vi "MCLB_FocusNameArray_Tests.vi"(11 "error in":errorcluster) -> (15 "error out":errorcluster)   [LabVIEW 2016, in "DronaTest.lvlib"]
uses:
  DronaTest.lvlib
  APIs/Stimulus/ControlValue/typedef/Name&Occurrence.ctl
  APIs/Stimulus/ControlValue/SetValueAuto.vi
  APIs/Stimulus/ControlValue/Controls/MC Listbox/SetValueByArrayName.vi
  APIs/Assert/AssertControlValue/Controls/MC Listbox/AssertValueByArrayName.vi
  <vilib>/addons/_JKI Toolkits/Caraya/classes/Assert/Assert Error.vi
  <vilib>/addons/_JKI Toolkits/Caraya/classes/Assert/Assert Equal Value_Variant.vi
  <vilib>/addons/_JKI Toolkits/Caraya/classes/Test/Test.lvclass
  Drona.lvlib
  <vilib>/SLL Toolkit/SLL Debug/SLL Debug.lvlib
  APIs/Stimulus/ControlValue/ControlValue.lvlib
  <vilib>/addons/_JKI Toolkits/Caraya/classes/Assert/Assert.lvclass
  APIs/Stimulus/ControlValue/Controls/MC Listbox/StimulusMCListbox.lvlib
  APIs/Assert/AssertControlValue/Controls/MC Listbox/AssertMCListbox.lvlib
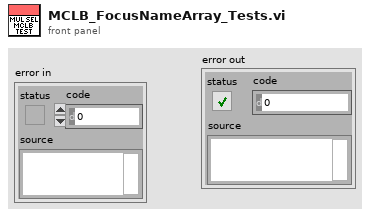
[diagram p1: front panel]
types:
  T1 = typedef "Drona.lvlib/ControlValue.lvlib/Name&Occurrence.ctl" = cluster{"ItemName":string, "Occurrence":i32}
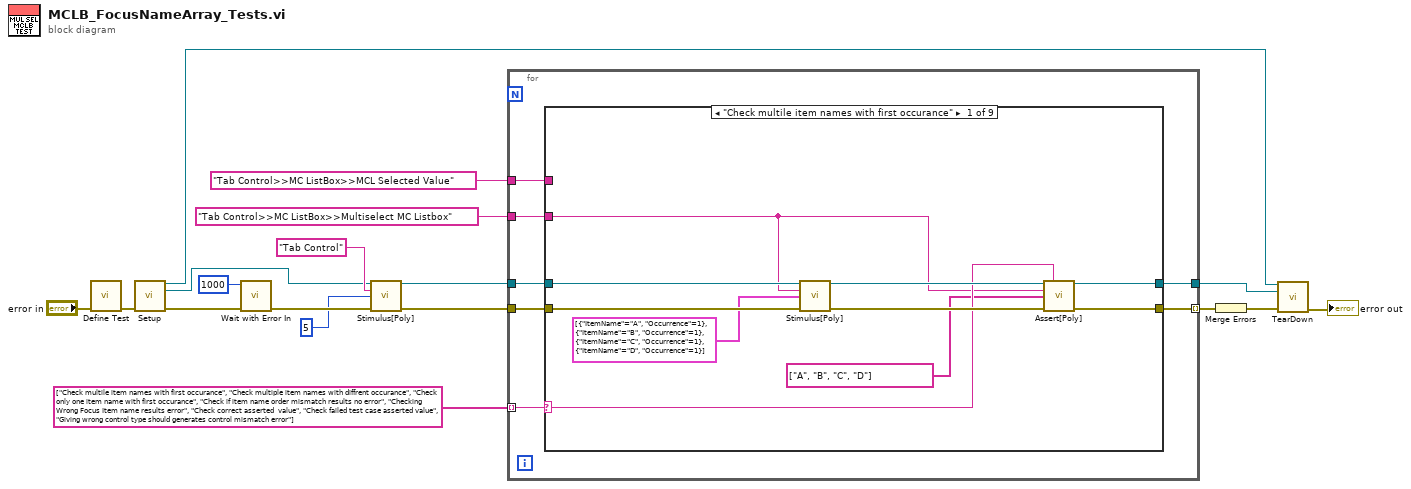
[diagram p0: block diagram]
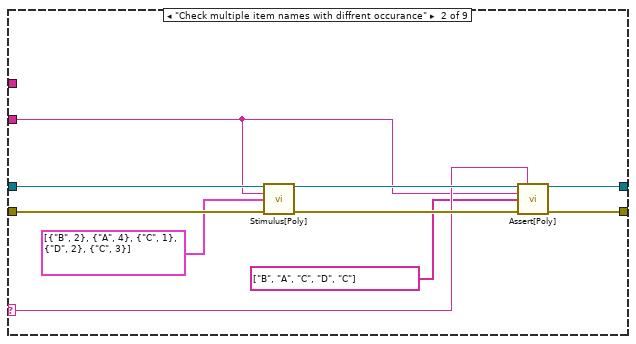
[diagram p2: hidden frame]
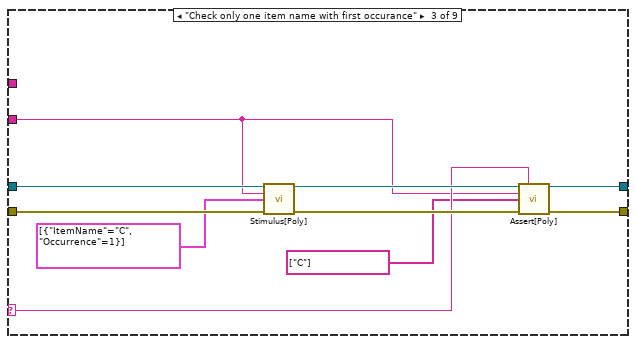
[diagram p3: hidden frame]
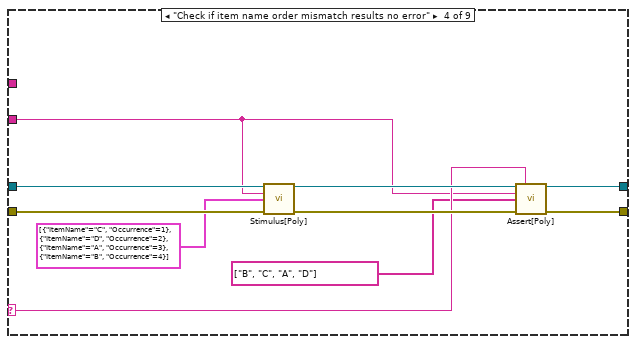
[diagram p4: hidden frame]
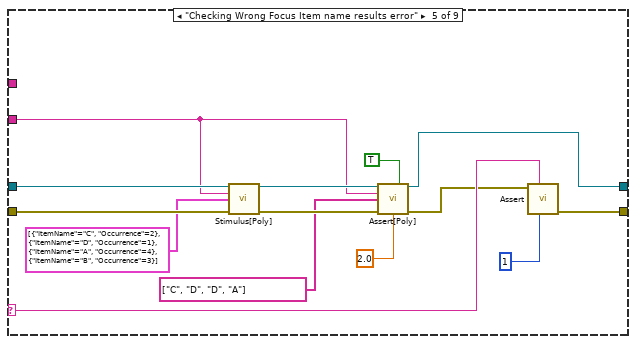
[diagram p5: hidden frame]
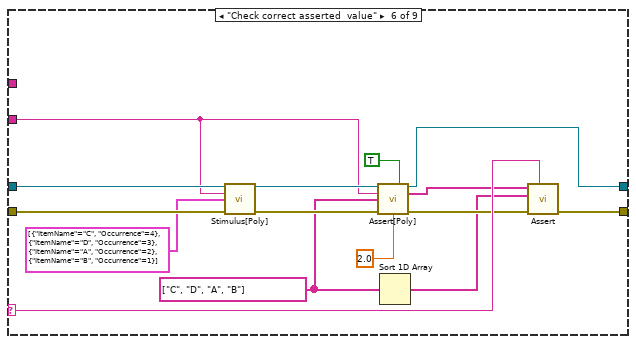
[diagram p6: hidden frame]
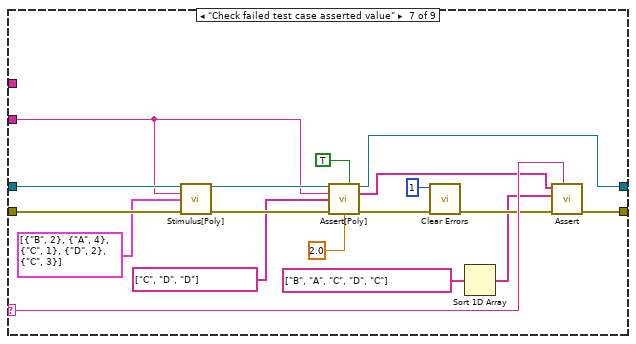
[diagram p7: hidden frame]
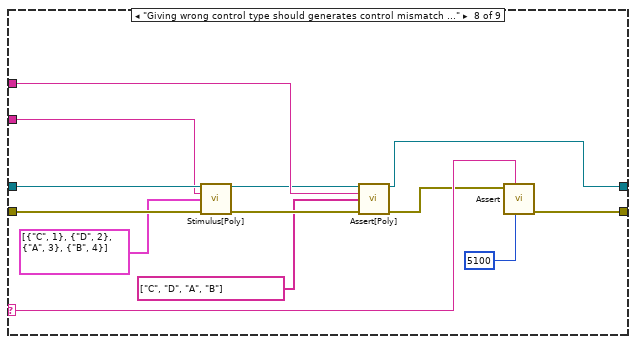
[diagram p8: hidden frame]
diagram:
  n1 = call <vilib>:"Define Test.vi"("error in (no error)"="error in") -> ("error out"=w7:errorcluster)  [unwired: 10 in]
  n2 = call "Setup.vi"("error in (no error)"=w7) -> ("Application Ref"=w3:refnum<vi>, "VI out"=w5:refnum<vi>, "error out"=w6:errorcluster)  [unwired: 12 in]
  n3 = call <vilib>:"Wait with Error In.vi"("error in (no error)"=w6, "milliseconds to wait"=u32 1000) -> ("error out"=w16:errorcluster)  [unwired: 9 in]
  n4 = call-poly "Stimulus[Poly].vi"("VI Reference In"=w5, "Control Path"="Tab Control", "Value (Signaling)"=5, "error in"=w16) -> ("VI Reference Out"=w12:refnum<vi>, "error out"=w15:errorcluster)  [unwired: 10 in]
  n5 = for {
    tunnel: w12 -> [w24]
    tunnel: "Tab Control>>MC ListBox>>Multiselect MC Listbox" ("Control Path") -> [w23]
    tunnel: "Tab Control>>MC ListBox>>MCL Selected Value" ("Control Path") -> [w22]
    tunnel: string[] ["Check multile item names with first occurance", "Check multiple item names with diffrent occurance", "Check only one item name with first occurance", "Check if item name order mismatch results no error", "Checking Wrong Focus Item name results error", "Check correct asserted  value", "Check failed test case asserted value", "Giving wrong control type should generates control mismatch error"] -> [w20] mode=indexing
    tunnel: [w19] -> w2
    tunnel: w15 -> [w25]
    tunnel: [w21] -> w8 mode=indexing
    n6 = case shown="\"Check multile item names with first occurance\"" w20 {
      selector: w20 -> [w29 w39 w49 w59 w78 w93 w111 w124 _]
      tunnel: w25 -> [w35 w45 w55 w65 w76 w92 w110 w119 w127]
      tunnel: w24 -> [w34 w44 w54 w64 w75 w91 w109 w117 w126]
      tunnel: w23 -> [w28 w38 w48 w58 w72 w88 w106 w115 _]
      tunnel: w22 -> [_ _ _ _ _ _ _ w121 _]
      tunnel: [w31 w41 w51 w61 w79 w94 w112 w125 w127] -> w21
      tunnel: [w30 w40 w50 w60 w71 w87 w105 w120 w126] -> w19
      frame "Check multile item names with first occurance" {
        n7 = call-poly "Stimulus[Poly].vi"("VI Reference In"=w34, "Control Path"=w28, "Name Array"=T1[] [{"ItemName"="A", "Occurrence"=1}, {"ItemName"="B", "Occurrence"=1}, {"ItemName"="C", "Occurrence"=1}, {"ItemName"="D", "Occurrence"=1}], "Error In"=w35) -> ("VI Reference Out"=w32:refnum<vi>, "Error Out"=w33:errorcluster)  [unwired: 10 in]
        n8 = call-poly "Assert[Poly].vi"("VI Reference In"=w32, "Test Label"=w29, "Control Path"=w28, "Focus Item Names"=string[] ["A", "B", "C", "D"], "Error In"=w33) -> ("VI Reference Out"=w30:refnum<vi>, "Error Out"=w31:errorcluster)  [unwired: 8 in, 1 out]
      }
      frame "Check multiple item names with diffrent occurance" {
        n9 = call-poly "Stimulus[Poly].vi"("VI Reference In"=w44, "Control Path"=w38, "Name Array"=T1[] [{"ItemName"="B", "Occurrence"=2}, {"ItemName"="A", "Occurrence"=4}, {"ItemName"="C", "Occurrence"=1}, {"ItemName"="D", "Occurrence"=2}, {"ItemName"="C", "Occurrence"=3}], "Error In"=w45) -> ("VI Reference Out"=w42:refnum<vi>, "Error Out"=w43:errorcluster)  [unwired: 10 in]
        n10 = call-poly "Assert[Poly].vi"("VI Reference In"=w42, "Test Label"=w39, "Control Path"=w38, "Focus Item Names"=string[] ["B", "A", "C", "D", "C"], "Error In"=w43) -> ("VI Reference Out"=w40:refnum<vi>, "Error Out"=w41:errorcluster)  [unwired: 8 in, 1 out]
      }
      frame "Check only one item name with first occurance" {
        n11 = call-poly "Stimulus[Poly].vi"("VI Reference In"=w54, "Control Path"=w48, "Name Array"=T1[] [{"ItemName"="C", "Occurrence"=1}], "Error In"=w55) -> ("VI Reference Out"=w52:refnum<vi>, "Error Out"=w53:errorcluster)  [unwired: 10 in]
        n12 = call-poly "Assert[Poly].vi"("VI Reference In"=w52, "Test Label"=w49, "Control Path"=w48, "Focus Item Names"=string[] ["C"], "Error In"=w53) -> ("VI Reference Out"=w50:refnum<vi>, "Error Out"=w51:errorcluster)  [unwired: 8 in, 1 out]
      }
      frame "Check if item name order mismatch results no error" {
        n13 = call-poly "Stimulus[Poly].vi"("VI Reference In"=w64, "Control Path"=w58, "Name Array"=T1[] [{"ItemName"="C", "Occurrence"=1}, {"ItemName"="D", "Occurrence"=2}, {"ItemName"="A", "Occurrence"=3}, {"ItemName"="B", "Occurrence"=4}], "Error In"=w65) -> ("VI Reference Out"=w62:refnum<vi>, "Error Out"=w63:errorcluster)  [unwired: 10 in]
        n14 = call-poly "Assert[Poly].vi"("VI Reference In"=w62, "Test Label"=w59, "Control Path"=w58, "Focus Item Names"=string[] ["B", "C", "A", "D"], "Error In"=w63) -> ("VI Reference Out"=w60:refnum<vi>, "Error Out"=w61:errorcluster)  [unwired: 8 in, 1 out]
      }
      frame "Checking Wrong Focus Item name results error" {
        n15 = call-poly "Stimulus[Poly].vi"("VI Reference In"=w75, "Control Path"=w72, "Name Array"=T1[] [{"ItemName"="C", "Occurrence"=2}, {"ItemName"="D", "Occurrence"=1}, {"ItemName"="A", "Occurrence"=4}, {"ItemName"="B", "Occurrence"=3}], "Error In"=w76) -> ("VI Reference Out"=w73:refnum<vi>, "Error Out"=w74:errorcluster)  [unwired: 10 in]
        n16 = call-poly "Assert[Poly].vi"("VI Reference In"=w73, "Assert Only? (F)"=TRUE, "Control Path"=w72, "Focus Item Names"=string[] ["C", "D", "D", "A"], "Error In"=w74, "Timeout(5 sec)"=2.0) -> ("VI Reference Out"=w71:refnum<vi>, "Error Out"=w70:errorcluster)  [unwired: 7 in, 1 out]
        n17 = call-poly <vilib>:"Assert.vi"("error code (1)"=1, "Label"=w78, "Error?"=w70) -> ("error out"=w79:errorcluster)  [unwired: 8 in]
      }
      frame "Check correct asserted  value" {
        w81 = string[] ["C", "D", "A", "B"] ("Focus Item Names")
        n18 = call-poly "Stimulus[Poly].vi"("VI Reference In"=w91, "Control Path"=w88, "Name Array"=T1[] [{"ItemName"="C", "Occurrence"=4}, {"ItemName"="D", "Occurrence"=3}, {"ItemName"="A", "Occurrence"=2}, {"ItemName"="B", "Occurrence"=1}], "Error In"=w92) -> ("VI Reference Out"=w89:refnum<vi>, "Error Out"=w90:errorcluster)  [unwired: 10 in]
        n19 = call-poly "Assert[Poly].vi"("VI Reference In"=w89, "Assert Only? (F)"=TRUE, "Control Path"=w88, "Focus Item Names"=w81, "Error In"=w90, "Timeout(5 sec)"=2.0) -> ("VI Reference Out"=w87:refnum<vi>, "Asserted Value"=w82:string[], "Error Out"=w83:errorcluster)  [unwired: 7 in]
        n20 = Sort 1D Array(array=w81) -> (sorted array=w80:string[])
        n21 = call-poly <vilib>:"Assert.vi"("Label"=w93, "error in (no error)"=w83, "Y"=w80, "X"=w82) -> ("error out"=w94:errorcluster)  [unwired: 7 in]
      }
      frame "Check failed test case asserted value" {
        n22 = call-poly "Stimulus[Poly].vi"("VI Reference In"=w109, "Control Path"=w106, "Name Array"=T1[] [{"ItemName"="B", "Occurrence"=2}, {"ItemName"="A", "Occurrence"=4}, {"ItemName"="C", "Occurrence"=1}, {"ItemName"="D", "Occurrence"=2}, {"ItemName"="C", "Occurrence"=3}], "Error In"=w110) -> ("VI Reference Out"=w107:refnum<vi>, "Error Out"=w108:errorcluster)  [unwired: 10 in]
        n23 = call-poly "Assert[Poly].vi"("VI Reference In"=w107, "Assert Only? (F)"=TRUE, "Control Path"=w106, "Focus Item Names"=string[] ["C", "D", "D"], "Error In"=w108, "Timeout(5 sec)"=2.0) -> ("VI Reference Out"=w105:refnum<vi>, "Asserted Value"=w99:string[], "Error Out"=w104:errorcluster)  [unwired: 7 in]
        n24 = call <vilib>:"Clear Errors.vi"("error in (no error)"=w104, "specific error code to clear (0: all)"=1) -> ("error out"=w101:errorcluster)  [unwired: 4 in, 1 out]
        n25 = Sort 1D Array(array=string[] ["B", "A", "C", "D", "C"] ("Focus Item Names")) -> (sorted array=w95:string[])
        n26 = call-poly <vilib>:"Assert.vi"("Label"=w111, "error in (no error)"=w101, "Y"=w95, "X"=w99) -> ("error out"=w112:errorcluster)  [unwired: 7 in]
      }
      frame "Giving wrong control type should generates control mismatch error" {
        n27 = call-poly "Stimulus[Poly].vi"("VI Reference In"=w117, "Control Path"=w115, "Name Array"=T1[] [{"ItemName"="C", "Occurrence"=1}, {"ItemName"="D", "Occurrence"=2}, {"ItemName"="A", "Occurrence"=3}, {"ItemName"="B", "Occurrence"=4}], "Error In"=w119) -> ("VI Reference Out"=w116:refnum<vi>, "Error Out"=w118:errorcluster)  [unwired: 10 in]
        n28 = call-poly "Assert[Poly].vi"("VI Reference In"=w116, "Control Path"=w121, "Focus Item Names"=string[] ["C", "D", "A", "B"], "Error In"=w118) -> ("VI Reference Out"=w120:refnum<vi>, "Error Out"=w122:errorcluster)  [unwired: 9 in, 1 out]
        n29 = call-poly <vilib>:"Assert.vi"("error code (1)"=5100, "Label"=w124, "Error?"=w122) -> ("error out"=w125:errorcluster)  [unwired: 8 in]
      }
      frame Default {
      }
    }
  }
  n30 = Merge Errors(w8) -> (w4:errorcluster)
  n31 = call "TearDown.vi"("Application Ref"=w3, "VI in"=w2, "error in (no error)"=w4) -> ("error out"=→"error out":errorcluster)  [unwired: 12 in]
